vi "Get Pixel at Cursor Location.vi"(8 "Error In":errorcluster, 9 "Mouse Coords in":T1, 11 "Image Refnum":refnum<vi>) -> (0 "Error Out":errorcluster, 1 "Pixel Coords out":T1, 3 "Valid coord":bool)   [LabVIEW 2021, in "Image.lvlib"]
uses:
  <vilib>/Utility/miscctls.llb/LVPoint32TypeDef.ctl
  Image.lvlib
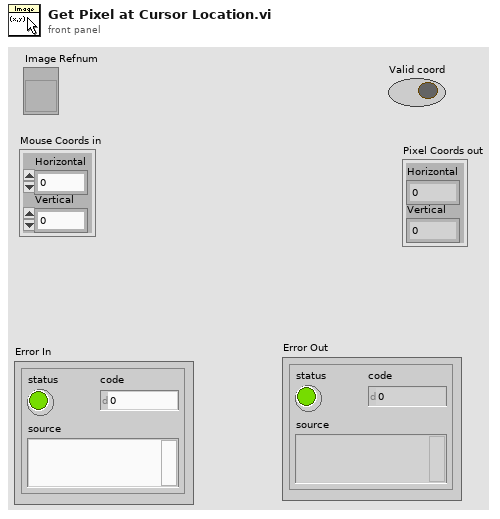
[diagram p1: front panel]
types:
  T1 = typedef "LVPoint32TypeDef.ctl" = cluster{"Horizontal":i32, "Vertical":i32}
  T2 = typedef "IMAQ Image.ctl" = refnum<image>
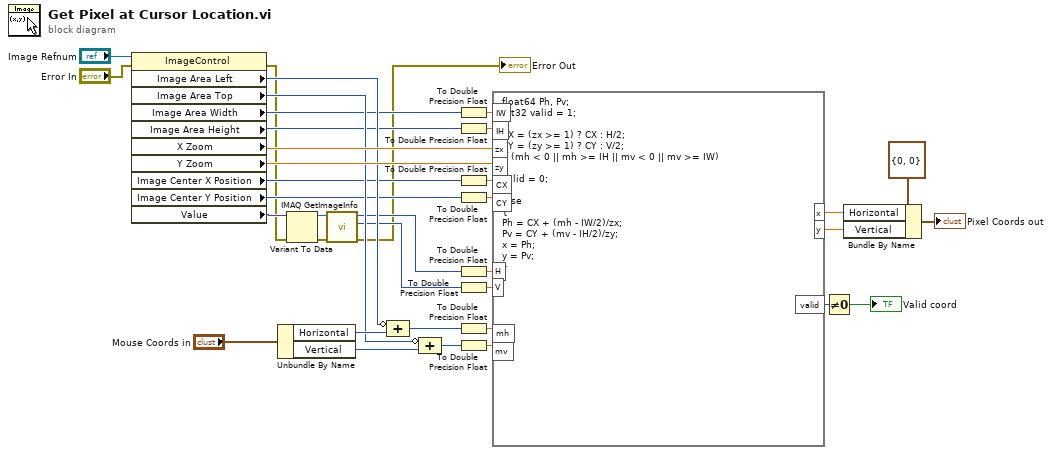
[diagram p0: block diagram]
diagram:
  n1 = property class="ImageControl"(reference="Image Refnum", error in="Error In") -> (error out=w2:errorcluster, "Image Area Left"=w22:i32, "Image Area Top"=w21:i32, "Image Area Width"=w20:u32, "Image Area Height"=w19:u32, "X Zoom"=w25:sgl, "Y Zoom"=w24:sgl, "Image Center X Position"=w18:u32, "Image Center Y Position"=w17:u32, "Value"=w8:variant)  [unwired: 1 out]
  n2 = Unbundle By Name("Mouse Coords in") -> ("Horizontal"=w35:i32, "Vertical"=w34:i32)
  n3 = Variant To Data(error in=w2, Variant=w8) -> (data=w7:T2, error out=w6:errorcluster)  [unwired: 1 in]
  n4 = call "IMAQ GetImageInfo"("error in (no error)"=w6, "Image"=w7) -> ("error out"=→"Error Out":errorcluster, "Y Resolution"=w4:i32, "X Resolution"=w5:i32)  [unwired: 2 in, 5 out]
  n5 = Compound Arithmetic op=ADD(invert w22, w35) -> (w29:i32)
  n6 = Compound Arithmetic op=ADD(invert w21, w34) -> (w28:i32)
  n7 = To Double Precision Float(number=w20) -> (double precision float=w16:dbl)
  n8 = To Double Precision Float(number=w19) -> (double precision float=w15:dbl)
  n9 = To Double Precision Float(number=w18) -> (double precision float=w14:dbl)
  n10 = To Double Precision Float(number=w17) -> (double precision float=w13:dbl)
  n11 = To Double Precision Float(number=w5) -> (double precision float=w12:dbl)
  n12 = To Double Precision Float(number=w4) -> (double precision float=w11:dbl)
  n13 = To Double Precision Float(number=w29) -> (double precision float=w10:dbl)
  n14 = To Double Precision Float(number=w28) -> (double precision float=w9:dbl)
  n15 = formula code="float64 Ph, Pv;\nint32 valid = 1;\n\nCX = (zx >= 1) ? CX : H/2;\nCY = (zy >= 1) ? CY : V/2;\nif (mh < 0 || mh >= IH || mv < 0 || mv >= IW)\n{\nvalid = 0;\n}\nelse\n{\nPh = CX + (mh - IW/2)/zx;\nPv = CY + (mv - IH/2)/zy;\nx = Ph;\ny = Pv;\n}"("H"=w12, "V"=w11, "mh"=w10, "mv"=w9, "zx"=w25, "zy"=w24, "IW"=w16, "IH"=w15, "CX"=w14, "CY"=w13) -> ("x"=w33:dbl, "y"=w32:dbl, "valid"=w27:i32)
  n16 = Not Equal To 0?(x=w27) -> (x != 0?=→"Valid coord":bool)
  n17 = Bundle By Name(cluster=T1 {"Horizontal"=0, "Vertical"=0} ("Pixel Coords out"), "Horizontal"=w33, "Vertical"=w32) -> (→"Pixel Coords out":T1)
